vi "SetImageType.vi"(8 "error in (no error)":errorcluster, 10 "Image Type (hex code)":u8 format="%.0x", 11 "CameraDemo in":refnum<class "CameraDemo.lvclass">) -> (0 "error out":errorcluster, 3 "CameraDemo out":refnum<class "CameraDemo.lvclass">)   [LabVIEW 2020, in "CameraI2COUSB.lvlib" / "CameraDemo.lvclass"]
uses:
  CameraDemo.lvclass
  CameraDemo.lvclass/CameraDemo.ctl
  Private/TypeDef/RegisterName.ctl
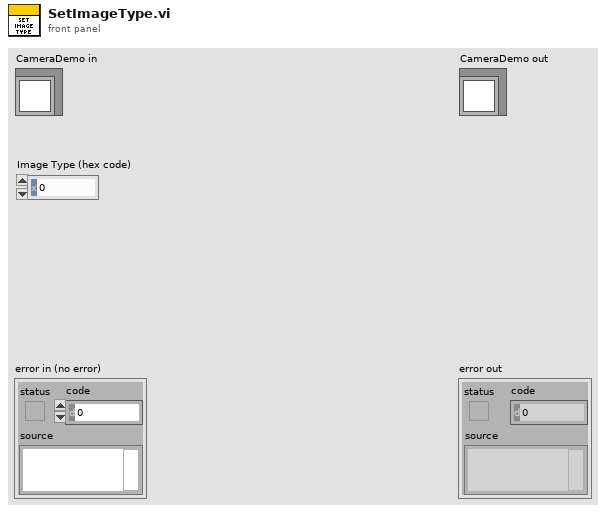
[diagram p1: front panel]
types:
  T1 = typedef "CameraI2COUSB.lvlib/CameraDemo.lvclass/RegisterName.ctl" = enum16{"Clock Rate", "Frame Rate", "Image Type", "Resolution", "Snap", "Start Streaming", "Stop Streaming"}
  T2 = typedef "CameraI2COUSB.lvlib/CameraDemo.lvclass/RegisterInfo.ctl" = cluster{"Address":u16, "Lenght":u32}
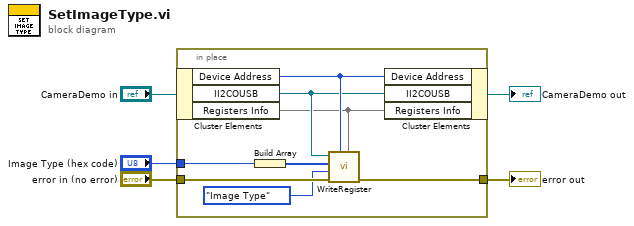
[diagram p0: block diagram]
diagram:
  n1 = in-place {
    in-place-border: "error in (no error)" -> [w13]
    in-place-border: "Image Type (hex code)" -> [w8]
    in-place-border: [w6] -> w3
    n2 = in-place-cluster #1("CameraDemo in") -> ("Device Address"=w12:u8, "II2COUSB"=w11:refnum<class "II2COUSB.lvclass">, "Registers Info"=w10:map{T1, T2})
    n3 = Build Array(w8) -> (w7:u8[])
    n4 = call "WriteRegister.vi"("Registers Info"=w10, "Device Address"=w12, "error in (no error)"=w13, "Register Name"=RegisterName."Image Type", "DATA"=w7, "II2COUSB"=w11) -> ("error out"=w6:errorcluster)  [unwired: 5 in]
    n5 = in-place-cluster #1("Device Address"=w12, "II2COUSB"=w11, "Registers Info"=w10) -> (→"CameraDemo out":refnum<class "CameraDemo.lvclass">)
  }
  "error out" <- w3
